vi "RTEH Error Notification.vi"(0 "Priority":i32, 1 "Command":T4, 5 "Classification":u32, 11 "Error to Send":cluster{"status":bool, "code":i32}, 12 "Configuration":T3) -> (3 "First Occurrence":timestamp, 4 "Priority Out":i32, 6 "Empty?":bool, 8 "Classification Out":u32, 10 "Transmitted Error":cluster{"status":bool, "code":i32}, 13 "Skipped?":bool=TRUE, 14 "Occurrences":i32, 15 "Internal Status":cluster{"Status":T1, "Error Code":i32})   [LabVIEW 2024]
uses:
  Controls/Shared/SEH Error Notification Command.ctl
  Controls/Shared/SEH Error Notification Config.ctl
  Controls/RTEH/RTEH Error Notification Data.ctl
  Controls/RTEH/RTEH Status Type.ctl
  Controls/Shared/SEH Transmit Error Function.ctl
panel:
  out "Read Ptrs":i32[](array[numeric])
  out "Array":T2[][](array[typedef])
  out "Codes":i32[][](array[numeric])
  out "Sizes":i32[](array[numeric])
  out "Write Ptrs":i32[](array[numeric])
  # "Debug"
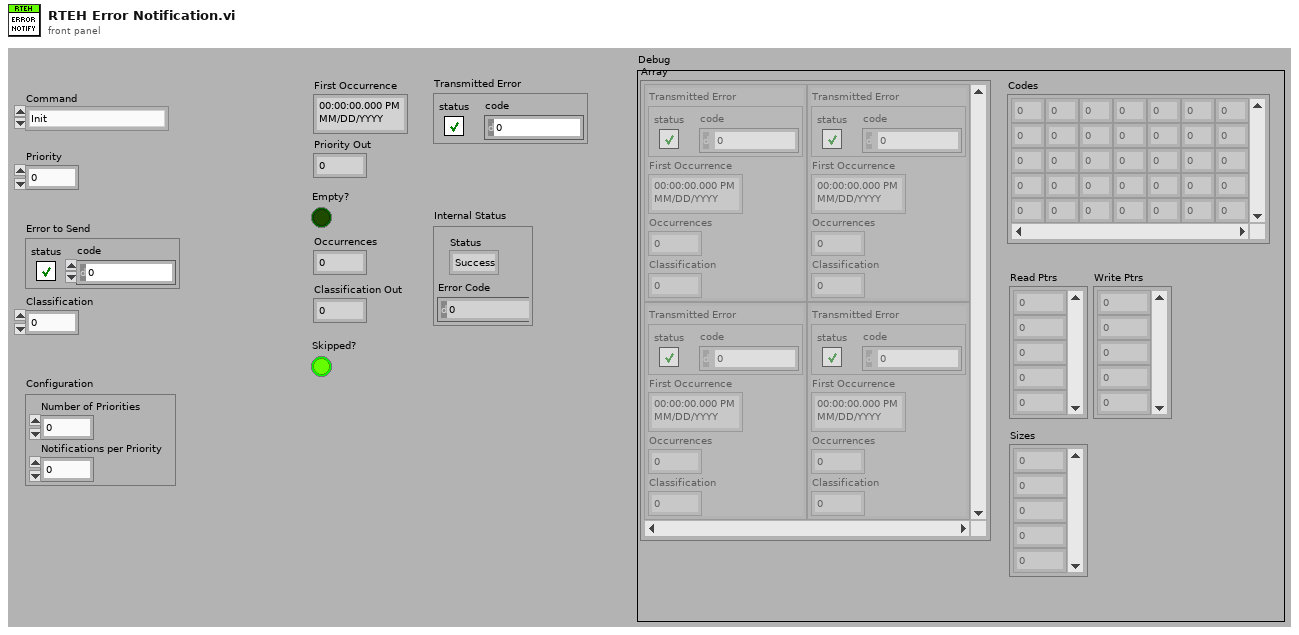
[diagram p1: front panel]
types:
  T1 = typedef "RTEH Status Type.ctl" = enum16{"Success", "Error", "Warning", "Skipped Notification"}
  T2 = typedef "RTEH Error Notification Data.ctl" = cluster{"Transmitted Error":cluster{"status":bool, "code":i32}, "First Occurrence":timestamp, "Occurrences":i32, "Classification":u32}
  T3 = typedef "SEH Error Notification Config.ctl" = cluster{"Number of Priorities":i32, "Notifications per Priority":i32}
  T4 = typedef "SEH Error Notification Command.ctl" = enum16{"Init", "Send Error", "Check Error", "Invalid Command"}
  T5 = typedef "SEH Transmit Error Function.ctl" = enum8{"Set", "Reset", "No Change"}
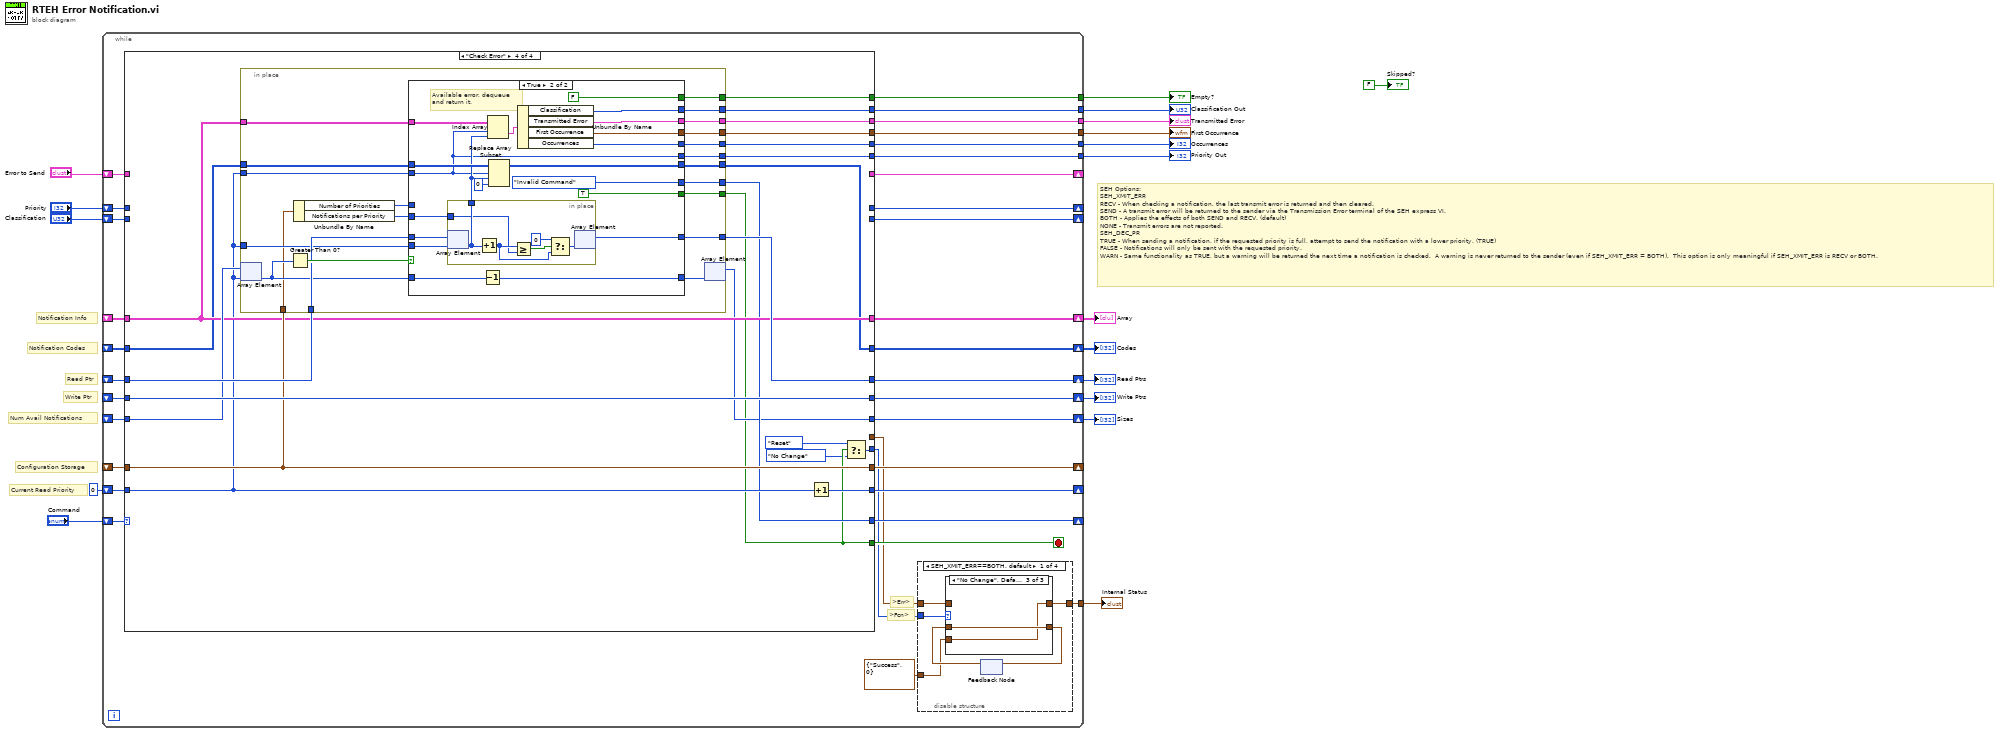
[diagram p0: block diagram]
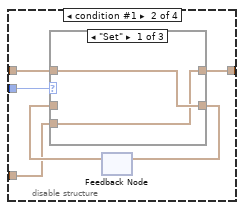
[diagram p4: hidden frame]
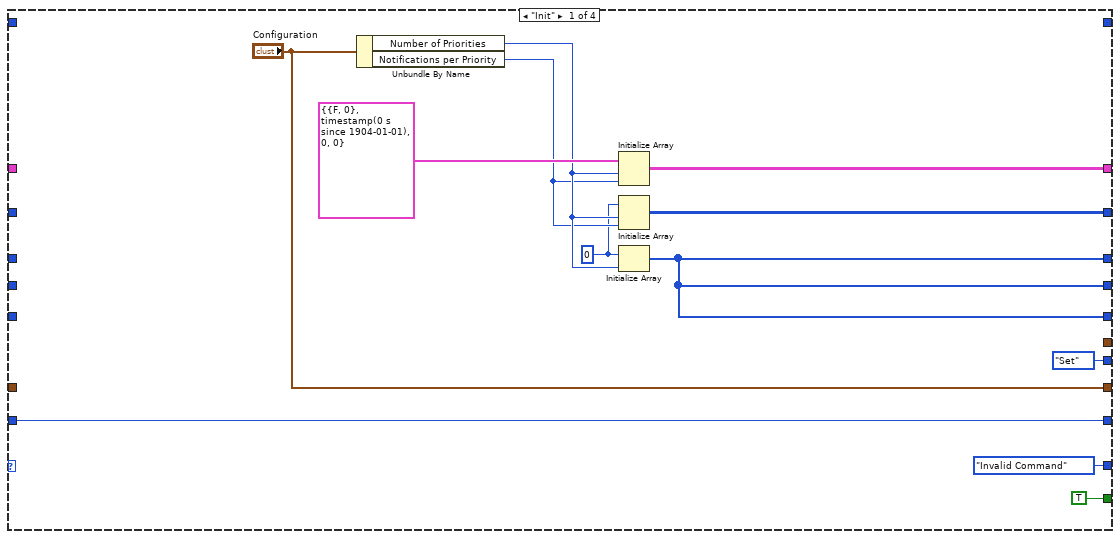
[diagram p9: hidden frame]
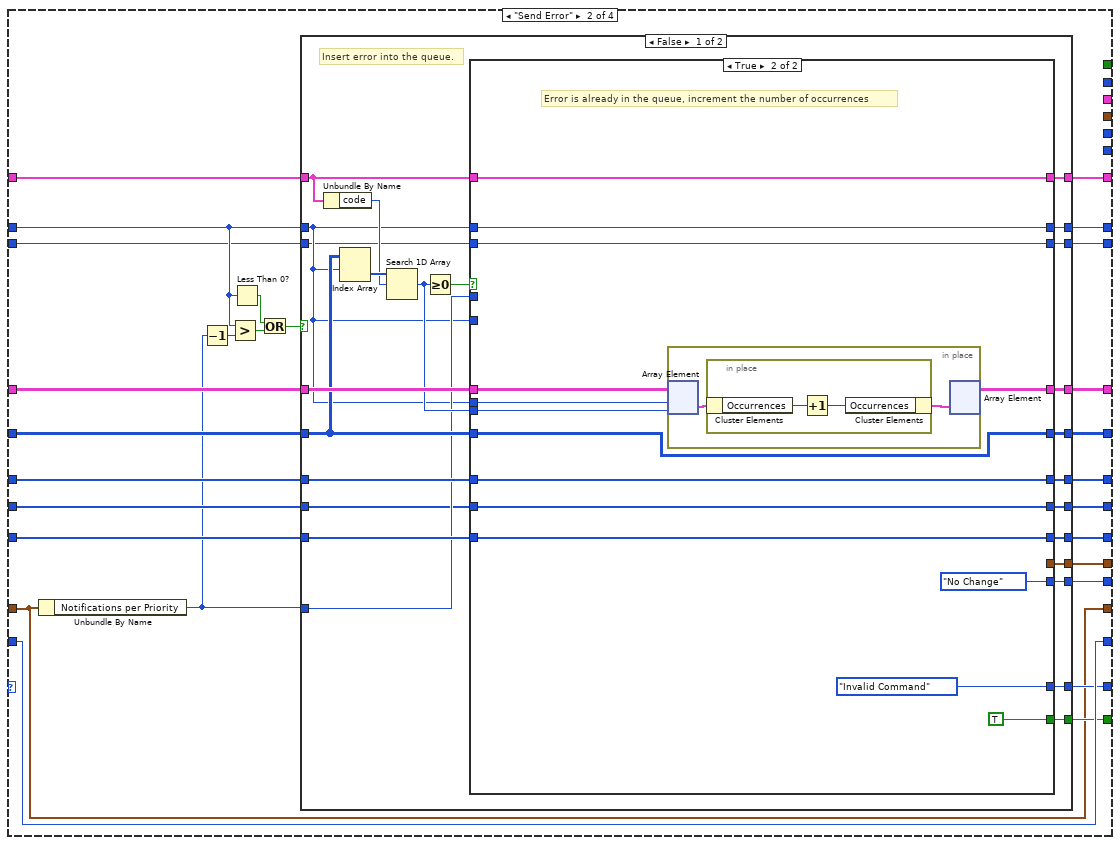
[diagram p10: hidden frame]
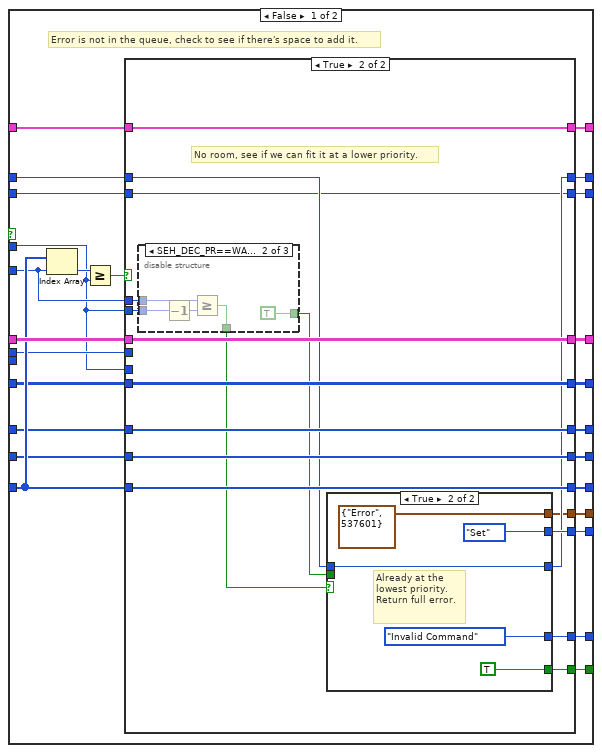
[diagram p11: hidden frame]
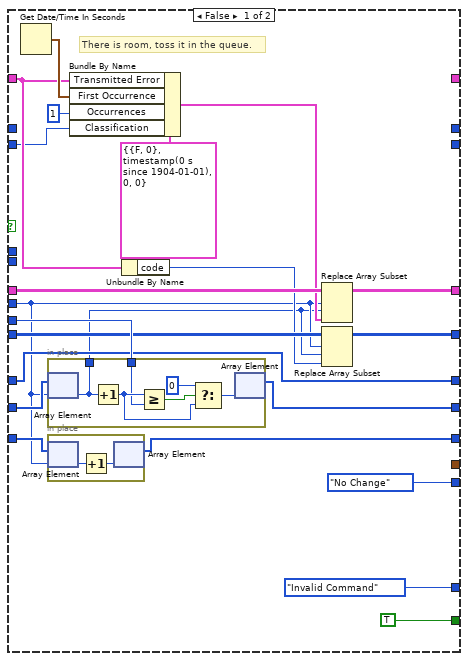
[diagram p12: hidden frame]
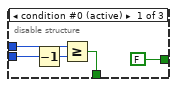
[diagram p13: hidden frame]
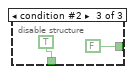
[diagram p14: hidden frame]
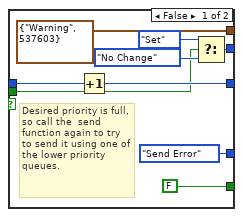
[diagram p15: hidden frame]
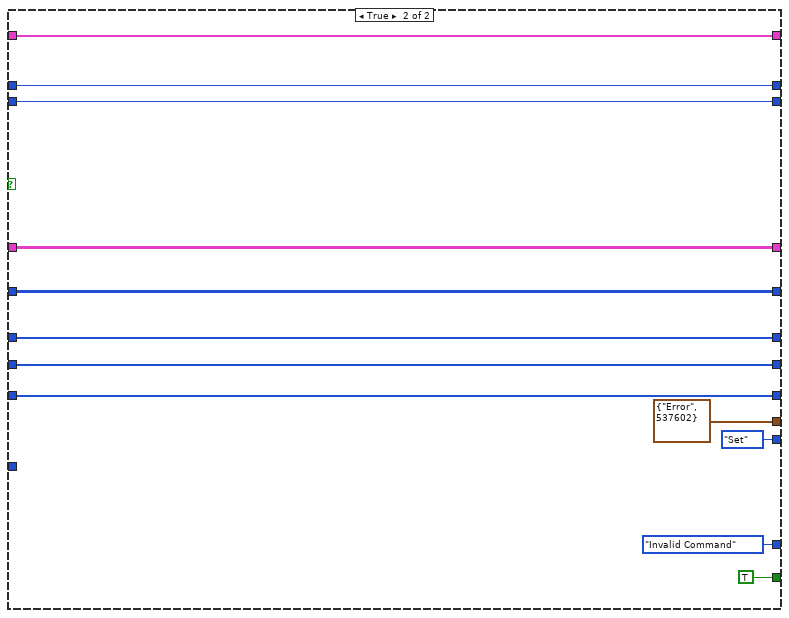
[diagram p16: hidden frame]
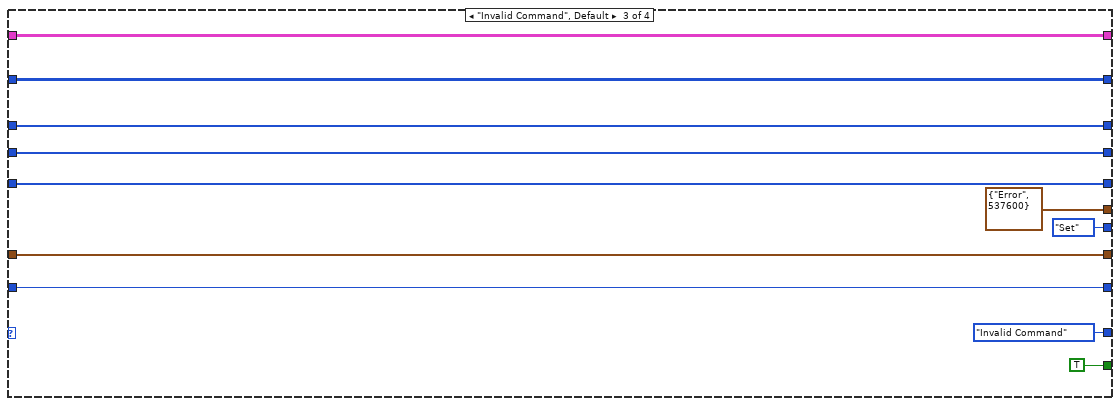
[diagram p17: hidden frame]
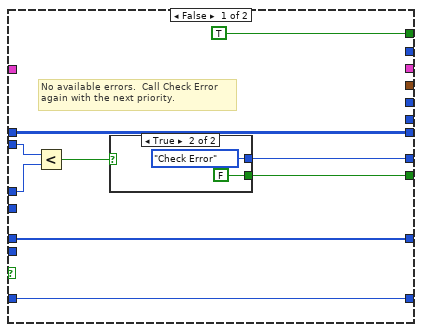
[diagram p18: hidden frame]
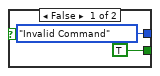
[diagram p19: hidden frame]
diagram:
  # "SEH Options:\nSEH_XMIT_ERR\nRECV - When checking a notification, the last transmit error is returned and then cleared.\nSEND - A transmit error will be returned to the sender via the Transmission Error terminal of the SEH express VI.\nBOTH - Applies the effects of both SEND and RECV. (default)\nNONE - Transmit errors are not reported.\nSEH_DEC_PR\nTRUE - When sending a notification, if the requested priority is full, attempt to send the notification with a lower priority. (TRUE)\nFALSE - Notifications will only be sent with the requested priority.\nWARN - Same functionality as TRUE, but a warning will be returned the next time a notification is checked.  A warning is never returned to the sender (even if SEH_XMIT_ERR = BOTH).  This option is only meaningful if SEH_XMIT_ERR is RECV or BOTH."
  # "Current Read Priority"
  # "Write Ptr"
  # "Configuration Storage"
  # "Notification Codes"
  # "Num Avail Notifications"
  # "Read Ptr"
  # "Notification Info"
  n1 = while {
    shift-right: [w50] -> w8
    shift-left: _ -> [w49]
    shift-right: [w48] -> w7
    shift-left: _ -> [w47]
    shift-right: [w46] -> w10
    shift-left: _ -> [w45]
    shift-right: [w44] -> _
    shift-left: _ -> [w43]
    shift-right: [w42] -> w9
    shift-left: _ -> [w41]
    shift-right: [w39] -> w11
    shift-left: _ -> [w38]
    shift-right: [w36] -> _
    shift-left: 0 -> [w37]
    shift-right: [w34] -> _
    shift-left: "Command" -> [w51]
    tunnel: [w33] -> w3
    tunnel: [w32] -> w14
    tunnel: [w31] -> w13
    tunnel: [w30] -> w12
    tunnel: [w29] -> w15
    shift-right: [w27] -> _
    shift-left: "Error to Send" -> [w40]
    shift-right: [w26] -> _
    shift-left: "Priority" -> [w28]
    tunnel: [w23] -> w5
    shift-right: [w20] -> _
    shift-left: "Classification" -> [w21]
    tunnel: [w19] -> w2
    stop <- w35 stop-if-true
    # ">Err>"
    # ">Fcn>"
    n2 = case shown="\"Check Error\"" w51 {
      tunnel: [w87 w112 w279 w295] -> w50
      tunnel: w49 -> [_ w115 w279 w295]
      tunnel: [w81 w110 w278 w297] -> w48
      tunnel: w47 -> [_ w111 w278 w299]
      tunnel: [w81 w108 w277 w285] -> w46
      tunnel: w45 -> [_ w109 w277 w296]
      tunnel: ["Configuration" w99 w276 w298] -> w44
      tunnel: w43 -> [_ w99 w276 w298]
      tunnel: [w83 w113 w275 w289] -> w42
      tunnel: w41 -> [_ w114 w275 w294]
      tunnel: w40 -> [_ w107 _ _]
      tunnel: [w81 w105 w274 w301] -> w39
      tunnel: w38 -> [_ w106 w274 w301]
      tunnel: w37 -> [w80 w104 w273 w293]
      tunnel: [w80 w104 w273 w300] -> w36
      tunnel: [TRUE w103 TRUE w284] -> w35
      tunnel: [SEH_Error_Notification_Command."Invalid Command" ("Command") w102 SEH_Error_Notification_Command."Invalid Command" ("Command") w286] -> w34
      tunnel: [_ _ _ w292] -> w33
      tunnel: [_ _ _ w291] -> w32
      tunnel: [_ _ _ w290] -> w31
      tunnel: [_ _ _ w288] -> w30
      tunnel: [_ _ _ w287] -> w29
      tunnel: w28 -> [_ w96 _ _]
      tunnel: [_ w101 _ _] -> w27
      tunnel: [_ w100 _ _] -> w26
      tunnel: [_ w92 cluster{"Status":T1, "Error Code":i32} {"Status"=enum."Error", "Error Code"=537600} ("Internal Status") _] -> w24
      tunnel: [SEH_Transmit_Error_Function."Set" w91 SEH_Transmit_Error_Function."Set" w281] -> w25
      tunnel: w21 -> [_ w90 _ _]
      tunnel: [_ w89 _ _] -> w20
      tunnel: [_ _ _ w280] -> w19
      frame "Init" {
        w84 = 0
        n3 = Unbundle By Name("Configuration") -> ("Number of Priorities"=w86:i32, "Notifications per Priority"=w85:i32)
        n4 = Initialize Array(T2 {"Transmitted Error"={"status"=FALSE, "code"=0}, "First Occurrence"=timestamp(0 s since 1904-01-01), "Occurrences"=0, "Classification"=0} ("Error Info"), w86, w85) -> (w87:T2[][])
        n5 = Initialize Array(w84, w86, w85) -> (w83:i32[][])
        n6 = Initialize Array(w84, w86) -> (w81:i32[])
      }
      frame "Send Error" {
        n7 = Unbundle By Name(w99) -> ("Notifications per Priority"=w98:i32)
        n8 = Decrement(x=w98) -> (x-1=w97:i32)
        n9 = Greater?(x=w96, y=w97) -> (0:w95:bool)
        n10 = Less Than 0?(x=w96) -> (x < 0?=w94:bool)
        n11 = Or(x=w94, y=w95) -> (x .or. y?=w93:bool)
        n12 = case shown="False" w93 {
          tunnel: w115 -> [w137 w261]
          tunnel: w114 -> [w135 w262]
          tunnel: [w134 w262] -> w113
          tunnel: [w133 w261] -> w112
          tunnel: w111 -> [w132 w263]
          tunnel: [w131 w263] -> w110
          tunnel: w109 -> [w130 w265]
          tunnel: [w129 w265] -> w108
          tunnel: w98 -> [w128 _]
          tunnel: w107 -> [w127 w268]
          tunnel: w106 -> [w126 w264]
          tunnel: [w125 w264] -> w105
          tunnel: [w124 TRUE] -> w103
          tunnel: [w123 SEH_Error_Notification_Command."Invalid Command" ("Command")] -> w102
          tunnel: [w122 w268] -> w101
          tunnel: w96 -> [w121 w260]
          tunnel: [w120 w260] -> w100
          tunnel: [w119 SEH_Transmit_Error_Function."Set"] -> w91
          tunnel: [w118 cluster{"Status":T1, "Error Code":i32} {"Status"=enum."Error", "Error Code"=537602} ("Internal Status")] -> w92
          tunnel: w90 -> [w117 w257]
          tunnel: [w116 w257] -> w89
          frame False {
            # "Insert error into the queue."
            n13 = Unbundle By Name(w127) -> ("code"=w139:i32)
            n14 = Index Array(array=w135, index (row)=w121) -> (element=w140:i32[])  [unwired: 1 in]
            n15 = Search 1D Array(1D array=w140, element=w139) -> (index of element=w136:i32)  [unwired: 1 in]
            n16 = Greater Or Equal To 0?(x=w136) -> (x >= 0?=w138:bool)
            n17 = case shown="True" w138 {
              tunnel: w137 -> [w163 w252]
              tunnel: w121 -> [w153 w251]
              tunnel: w136 -> [_ w250]
              tunnel: w135 -> [w156 w249]
              tunnel: [w155 w249] -> w134
              tunnel: [w162 w248] -> w133
              tunnel: w132 -> [w158 w247]
              tunnel: [w157 w247] -> w131
              tunnel: w130 -> [w160 w246]
              tunnel: [w159 w246] -> w129
              tunnel: [w161 SEH_Transmit_Error_Function."No Change"] -> w119
              tunnel: w128 -> [w144 _]
              tunnel: w127 -> [w154 w243]
              tunnel: w126 -> [w152 w245]
              tunnel: [w151 w245] -> w125
              tunnel: w121 -> [w148 _]
              tunnel: [w150 TRUE] -> w124
              tunnel: [w149 SEH_Error_Notification_Command."Invalid Command" ("Command")] -> w123
              tunnel: [w147 w243] -> w122
              tunnel: w121 -> [w146 w242]
              tunnel: [w145 w242] -> w120
              tunnel: [w143 _] -> w118
              tunnel: w117 -> [w142 w239]
              tunnel: [w141 w239] -> w116
              frame False {
                # "Error is not in the queue, check to see if there's space to add it."
                n18 = Index Array(array=w160, index=w148) -> (element=w165:i32)
                n19 = Greater Or Equal?(x=w165, y=w144) -> (x >= y?=w164:bool)
                n20 = case shown="True" w164 {
                  tunnel: w163 -> [w187 w212]
                  tunnel: [w186 w212] -> w162
                  tunnel: [SEH_Transmit_Error_Function."No Change" w211] -> w161
                  tunnel: w160 -> [w181 w210]
                  tunnel: [w180 w210] -> w159
                  tunnel: [w176 w209] -> w157
                  tunnel: w158 -> [w176 w209]
                  tunnel: w156 -> [w175 w208]
                  tunnel: [w174 w208] -> w155
                  tunnel: w154 -> [w173 w202]
                  tunnel: w153 -> [w171 _]
                  tunnel: w152 -> [w178 w207]
                  tunnel: [w179 w207] -> w151
                  tunnel: w144 -> [w177 _]
                  tunnel: [TRUE w206] -> w150
                  tunnel: [SEH_Error_Notification_Command."Invalid Command" ("Command") w205] -> w149
                  tunnel: w148 -> [_ w204]
                  tunnel: w144 -> [_ w199]
                  tunnel: [_ w202] -> w147
                  tunnel: w146 -> [_ w201]
                  tunnel: [_ w200] -> w145
                  tunnel: [_ w198] -> w143
                  tunnel: w142 -> [w166 w196]
                  tunnel: [_ w196] -> w141
                  frame False {
                    # "There is room, toss it in the queue."
                    n21 = Get Date/Time In Seconds() -> (seconds since 1Jan1904=w182:timestamp)
                    n22 = in-place {
                      in-place-border: [w189] -> w170
                      in-place-border: w177 -> [w188]
                      n23 = in-place-array #1(w178, w171) -> (w189:i32)
                      n24 = Increment(x=w189) -> (x+1=w192:i32)
                      n25 = Greater Or Equal?(x=w192, y=w188) -> (x >= y?=w193:bool)
                      n26 = Select(t=0, s=w193, f=w192) -> (s? t:f=w190:i32)
                      n27 = in-place-array #1(w190) -> (w179:i32[])  [unwired: 1 out]
                    }
                    n28 = in-place {
                      n29 = in-place-array #2(w181, w171) -> (w195:i32)
                      n30 = Increment(x=w195) -> (x+1=w194:i32)
                      n31 = in-place-array #2(w194) -> (w180:i32[])  [unwired: 1 out]
                    }
                    n32 = Bundle By Name(cluster=T2 {"Transmitted Error"={"status"=FALSE, "code"=0}, "First Occurrence"=timestamp(0 s since 1904-01-01), "Occurrences"=0, "Classification"=0} ("Error Info"), "Transmitted Error"=w173, "First Occurrence"=w182, "Occurrences"=1, "Classification"=w166) -> (w183:T2)
                    n33 = Unbundle By Name(w173) -> ("code"=w172:i32)
                    n34 = Replace Array Subset(array=w187, new element=w183, index (row)=w171, index (col)=w170) -> (w186:T2[][])
                    n35 = Replace Array Subset(array=w175, new element=w172, index (row)=w171, index (col)=w170) -> (w174:i32[][])
                  }
                  frame True {
                    # "No room, see if we can fit it at a lower priority."
                    n36 = disable-structure shown="SEH_DEC_PR==WARN" {
                      disable-tunnel: w204 -> [w217 w222 _]
                      disable-tunnel: [w216 w221 TRUE] -> w203
                      disable-tunnel: w199 -> [w215 w220 _]
                      disable-tunnel: [FALSE TRUE FALSE] -> w197
                      frame condition #0 (active) {
                        n37 = Decrement(x=w215) -> (x-1=w214:i32)
                        n38 = Greater Or Equal?(x=w217, y=w214) -> (x >= y?=w216:bool)
                      }
                      frame condition #1 {
                        n39 = Decrement(x=w220) -> (x-1=w219:i32)
                        n40 = Greater Or Equal?(x=w222, y=w219) -> (x >= y?=w221:bool)
                      }
                      frame condition #2 {
                      }
                    }
                    n41 = case shown="True" w203 {
                      tunnel: [w228 SEH_Transmit_Error_Function."Set"] -> w211
                      tunnel: [FALSE TRUE] -> w206
                      tunnel: [SEH_Error_Notification_Command."Send Error" ("Command") SEH_Error_Notification_Command."Invalid Command" ("Command")] -> w205
                      tunnel: w201 -> [w233 w236]
                      tunnel: [w232 w236] -> w200
                      tunnel: [cluster{"Status":T1, "Error Code":i32} {"Status"=enum."Warning", "Error Code"=537603} ("Internal Status") cluster{"Status":T1, "Error Code":i32} {"Status"=enum."Error", "Error Code"=537601} ("Internal Status")] -> w198
                      tunnel: w197 -> [w227 _]
                      frame False {
                        # "Desired priority is full, so call the  send function again to try to send it using one of the lower priority queues."
                        n42 = Increment(x=w233) -> (x+1=w232:i32)
                        n43 = Select(t=SEH_Transmit_Error_Function."Set", s=w227, f=SEH_Transmit_Error_Function."No Change") -> (s? t:f=w228:T5)
                      }
                      frame True {
                        # "Already at the lowest priority.\nReturn full error."
                      }
                    }
                  }
                }
              }
              frame True {
                # "Error is already in the queue, increment the number of occurrences"
                # "Error is already in the queue, increase # of occurrences"
                n44 = in-place {
                  n45 = in-place-array #3(w252, w251, w250) -> (w254:T2)
                  n46 = in-place {
                    n47 = in-place-cluster #4(w254) -> ("Occurrences"=w256:i32)
                    n48 = Increment(x=w256) -> (x+1=w255:i32)
                    n49 = in-place-cluster #4("Occurrences"=w255) -> (w253:T2)
                  }
                  n50 = in-place-array #3(w253) -> (w248:T2[][])  [unwired: 2 out]
                }
              }
            }
          }
          frame True {
          }
        }
      }
      frame "Invalid Command", Default {
      }
      frame "Check Error" {
        n51 = in-place {
          in-place-border: w299 -> [w321]
          in-place-border: w298 -> [w305]
          in-place-border: [w320] -> w297
          in-place-border: w293 -> [w319]
          in-place-border: w295 -> [w315]
          in-place-border: w294 -> [w316]
          in-place-border: w293 -> [w314]
          in-place-border: [w313] -> w292
          in-place-border: [w312] -> w291
          in-place-border: [w311] -> w290
          in-place-border: [w310] -> w289
          in-place-border: [w309] -> w288
          in-place-border: [w308] -> w287
          in-place-border: [w307] -> w286
          in-place-border: [w306] -> w284
          in-place-border: [w302] -> w280
          n52 = in-place-array #5(w296, w293) -> (w318:i32)
          n53 = Greater Than 0?(x=w318) -> (x > 0?=w322:bool)
          n54 = Unbundle By Name(w305) -> ("Number of Priorities"=w303:i32, "Notifications per Priority"=w304:i32)
          n55 = case shown="True" w322 {
            tunnel: w321 -> [w330 w355]
            tunnel: [w330 w354] -> w320
            tunnel: w319 -> [_ w353]
            tunnel: w318 -> [w331 w352]
            tunnel: [w331 w351] -> w317
            tunnel: w316 -> [w329 w350]
            tunnel: w315 -> [_ w348]
            tunnel: w314 -> [w325 w341]
            tunnel: [_ w345] -> w313
            tunnel: [_ w344] -> w312
            tunnel: [_ w343] -> w311
            tunnel: [w329 w342] -> w310
            tunnel: [_ w341] -> w309
            tunnel: [TRUE FALSE] -> w308
            tunnel: [w327 SEH_Error_Notification_Command."Invalid Command" ("Command")] -> w307
            tunnel: [w326 TRUE] -> w306
            tunnel: w304 -> [_ w337]
            tunnel: w303 -> [w324 _]
            tunnel: [_ w336] -> w302
            frame False {
              # "No available errors.  Call Check Error \nagain with the next priority."
              n56 = Less?(x=w325, y=w324) -> (x < y?=w323:bool)
              n57 = case shown="True" w323 {
                tunnel: [SEH_Error_Notification_Command."Invalid Command" ("Command") SEH_Error_Notification_Command."Check Error" ("Command")] -> w327
                tunnel: [TRUE FALSE] -> w326
                frame False {
                }
                frame True {
                }
              }
            }
            frame True {
              # "Available error, dequeue \nand return it."
              n58 = in-place {
                in-place-border: [w357] -> w347
                in-place-border: w337 -> [w356]
                n59 = in-place-array #6(w355, w353) -> (w357:i32)
                n60 = Increment(x=w357) -> (x+1=w360:i32)
                n61 = Greater Or Equal?(x=w360, y=w356) -> (x >= y?=w361:bool)
                n62 = Select(t=0, s=w361, f=w360) -> (s? t:f=w358:i32)
                n63 = in-place-array #6(w358) -> (w354:i32[])  [unwired: 1 out]
              }
              n64 = Decrement(x=w352) -> (x-1=w351:i32)
              n65 = Index Array(array=w348, index (row)=w341, index (col)=w347) -> (element=w346:T2)
              n66 = Replace Array Subset(array=w350, new element=0 ("new element/subarray"), index (row)=w341, index (col)=w347) -> (w342:i32[][])
              n67 = Unbundle By Name(w346) -> ("Classification"=w336:u32, "Transmitted Error"=w345:cluster{"status":bool, "code":i32}, "First Occurrence"=w344:timestamp, "Occurrences"=w343:i32)
            }
          }
          n68 = in-place-array #5(w317) -> (w285:i32[])  [unwired: 1 out]
        }
        n69 = Increment(x=w293) -> (x+1=w300:i32)
        n70 = Select(t=SEH_Transmit_Error_Function."Reset", s=w284, f=SEH_Transmit_Error_Function."No Change") -> (s? t:f=w281:T5)
      }
    }
    n71 = disable-structure shown="SEH_XMIT_ERR==BOTH, default" {
      disable-tunnel: w24 -> [w56 w67 w75 _]
      disable-tunnel: w25 -> [w57 w68 _ _]
      disable-tunnel: [w53 w64 w75 w76] -> w23
      disable-tunnel: cluster{"Status":T1, "Error Code":i32} {"Status"=enum."Success", "Error Code"=0} ("Internal Status") -> [w52 w63 _ w76]
      frame condition #0 (active) {
        n72 = feedback #7() -> (w54:cluster{"Status":T1, "Error Code":i32})  [unwired: 1 in]
        n73 = case shown="\"No Change\", Default" w57 {
          tunnel: w56 -> [w58 _ _]
          tunnel: w52 -> [_ w60 w61]
          tunnel: [w58 w60 w62] -> w55
          tunnel: w54 -> [_ w59 w62]
          tunnel: [w58 w59 w61] -> w53
          frame "Set" {
          }
          frame "Reset" {
          }
          frame "No Change", Default {
          }
        }
        n74 = feedback-in #7(w55) -> ()
      }
      frame condition #1 {
        n75 = feedback #8() -> (w65:cluster{"Status":T1, "Error Code":i32})  [unwired: 1 in]
        n76 = case shown="\"Set\"" w68 {
          tunnel: w67 -> [w70 _ _]
          tunnel: w63 -> [w69 w72 w73]
          tunnel: [w70 w72 w74] -> w66
          tunnel: w65 -> [_ w71 w74]
          tunnel: [w69 w71 w73] -> w64
          frame "Set" {
          }
          frame "Reset" {
          }
          frame "No Change", Default {
          }
        }
        n77 = feedback-in #8(w66) -> ()
      }
      frame condition #2 {
      }
      frame condition #3 {
      }
    }
  }
  "Empty?" <- w15
  "Priority Out" <- w12
  "First Occurrence" <- w14
  "Occurrences" <- w13
  "Transmitted Error" <- w3
  "Write Ptrs" <- w11
  "Sizes" <- w10
  "Codes" <- w9
  "Array" <- w8
  "Read Ptrs" <- w7
  "Internal Status" <- w5
  "Classification Out" <- w2
  "Skipped?" <- FALSE ("Skipped?")
